vi "Test_WriteItem_FloatKey_ReadItem_ItemReturned.vi"(8 "error in (no error)":errorcluster, 11 "TestCase in":refnum<class "TestComposedLookupTable.lvclass">) -> (0 "error out":errorcluster, 3 "TestCase out":refnum<class "TestComposedLookupTable.lvclass">)   [LabVIEW 2017, in "TestComposedLookupTable.lvclass"]
uses:
  TestComposedLookupTable.lvclass
  Source/LookupTable/LookupTable.lvclass/LookupTable.ctl
  de331345-f2dc-4322-a95c-a178be91e42b.vi
  d0b264f1-442b-48e7-b5c6-30e921ae893d.vi
  Source/LookupTable/Read Table Reference.vi
  de331345-f2dc-4322-a95c-a178be91e42b.vi/acc272e5-fd85-4fbb-b545-457fe05d68bd.vi
  d0b264f1-442b-48e7-b5c6-30e921ae893d.vi/cb16d91f-7dc1-4934-8d61-48f87877f0ed.vi
  Source/LookupTable/LookupTable.lvclass
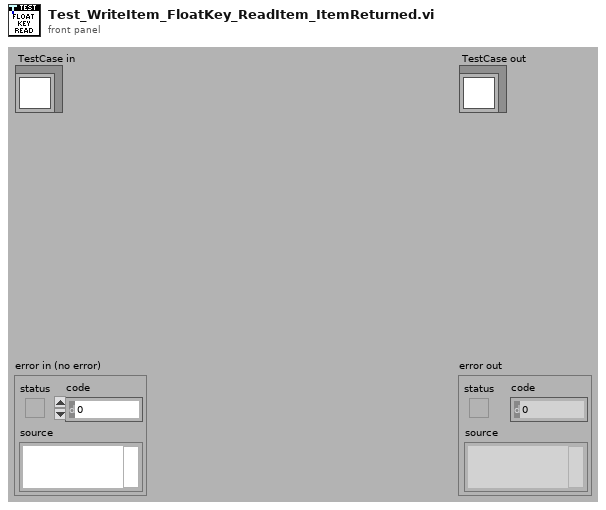
[diagram p1: front panel]
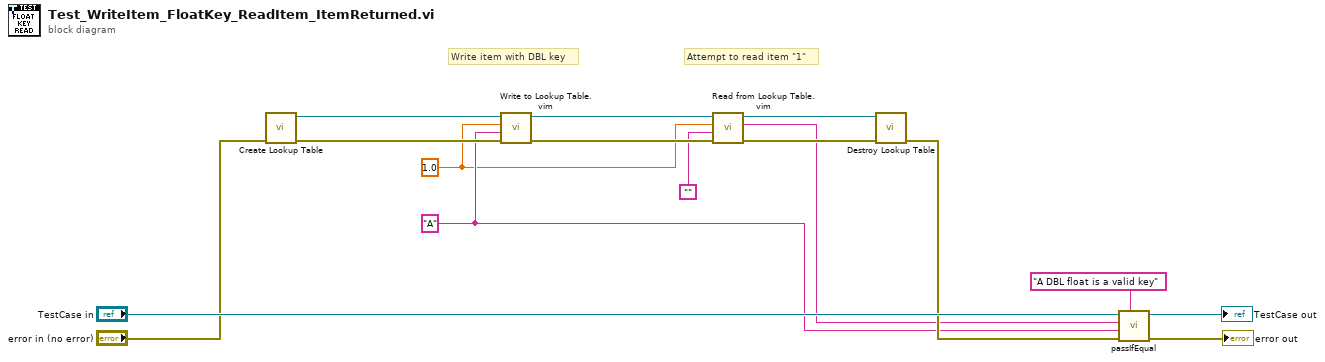
[diagram p0: block diagram]
diagram:
  w1 = 1.0
  w4 = "A" ("Item Name")
  # "Attempt to read item \"1\""
  # "Write item with DBL key"
  n1 = call "Create Lookup Table.vi"("error in (no error)"="error in (no error)") -> ("error out"=w16:errorcluster, "LookupTable Reference"=w8:refnum<data-value>)  [unwired: 9 in]
  n2 = call "Write to Lookup Table.vim"("error in (no error)"=w16, "Item"=w4, "Item Name"=w1, "LookupTable Reference"=w8) -> ("error out"=w10:errorcluster, "LookupTable Reference Out"=w6:refnum<data-value>)  [unwired: 5 in, 1 out]
  n3 = call "Read from Lookup Table.vim"("error in (no error)"=w10, "Type"="", "Item Name"=w1, "LookupTable Reference"=w6) -> ("error out"=w7:errorcluster, "Value"=w5:string, "LookupTable Reference Out"=w11:refnum<data-value>)  [unwired: 4 in, 1 out]
  n4 = call "Destroy Lookup Table.vi"("error in (no error)"=w7, "LookupTable Reference"=w11) -> ("error out"=w9:errorcluster)  [unwired: 9 in]
  n5 = call-dynamic "passIfEqual.vi"("custom report message (\"\")"="A DBL float is a valid key" ("message (\"\")"), "error in (no error)"=w9, "y"=w4, "x"=w5, "TestCase in"="TestCase in") -> ("error out"=→"error out":errorcluster, "TestCase out"=→"TestCase out":refnum<class "TestComposedLookupTable.lvclass">)  [unwired: 5 in]
